vi "Edit waveform read from MDO.vi"() -> ()   [LabVIEW 2020]
uses:
  <vilib>/Utility/file.llb/Write Delimited Spreadsheet (DBL).vi
panel:
  in  "file (use dialog) in":path
  out "Array":dbl[][](array[numeric])
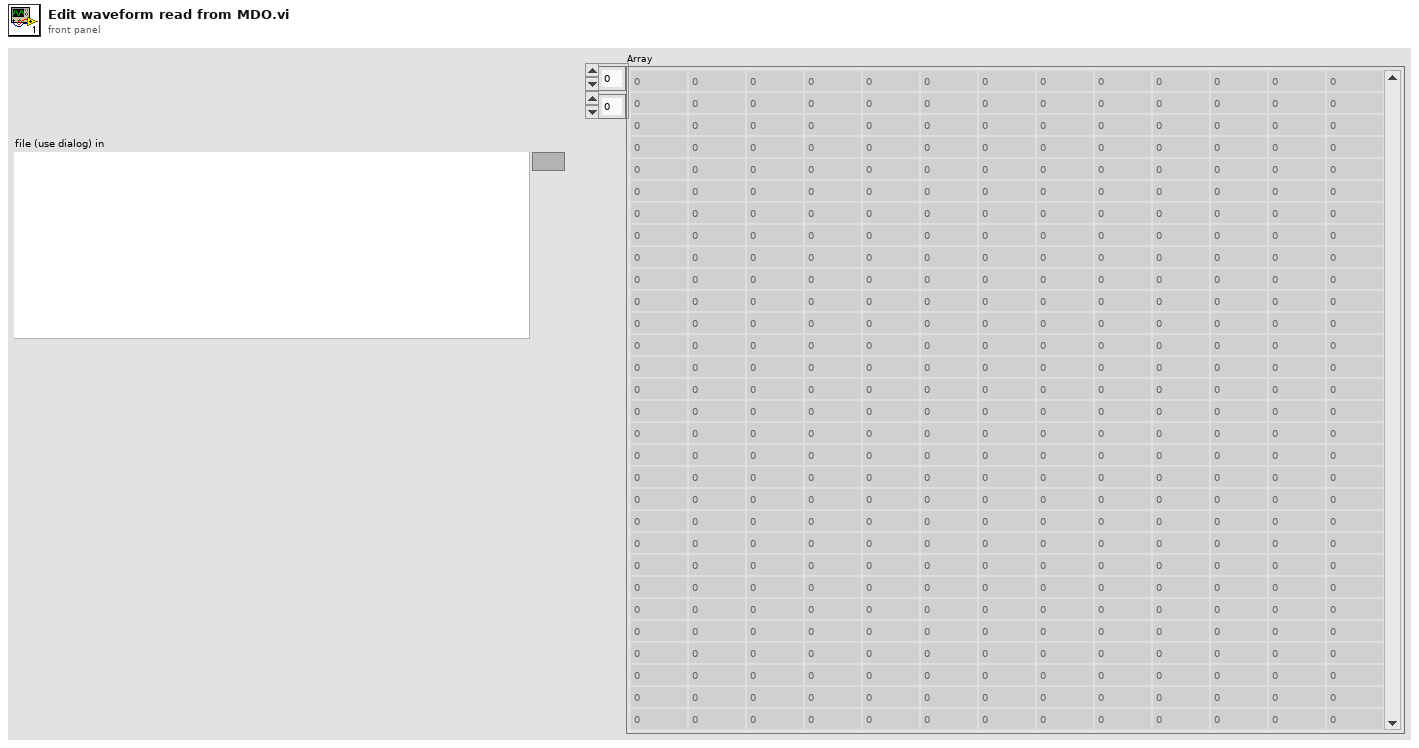
[diagram p1: front panel]
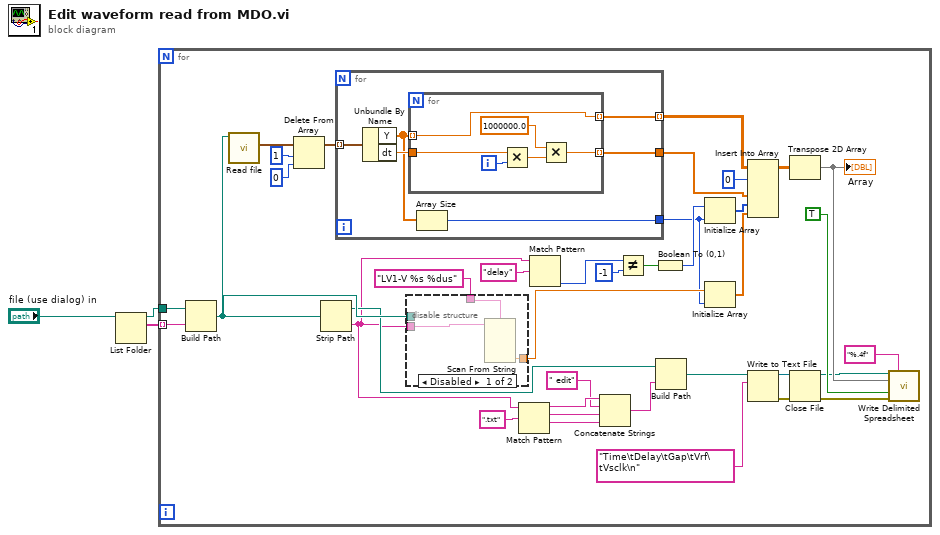
[diagram p0: block diagram]
diagram:
  n1 = List Folder(path="file (use dialog) in") -> (path out=w2:path, filenames=w1:string[])  [unwired: 3 in, 2 out]
  n2 = for {
    tunnel: w2 -> [w16]
    tunnel: w1 -> [w15] mode=indexing
    n3 = Build Path(base path=w16, name or relative path=w15) -> (appended path=w14:path)
    n4 = call "Read file.vi"("file (use dialog) in"=w14) -> ("Waveform Array"=w37:waveform(dbl)[])  [unwired: 7 in, 3 out]
    n5 = Delete From Array(array=w37, length=1, index=0) -> (array with subset deleted=w36:waveform(dbl)[])  [unwired: 1 out]
    n6 = Strip Path(path=w14) -> (stripped path=w5:path, name=w4:string)
    n7 = for {
      tunnel: w36 -> [w50] mode=indexing
      tunnel: [w48] -> w41 mode=indexing
      tunnel: [w47] -> w40
      tunnel: [w45] -> w8
      n8 = Unbundle By Name(w50) -> ("Y"=w46:dbl[], "dt"=w49:dbl)
      n9 = for {
        tunnel: w46 -> [w54] mode=indexing
        tunnel: w49 -> [w55]
        tunnel: [w54] -> w48 mode=indexing
        tunnel: [w51] -> w47 mode=indexing
        i -> [w56]
        n10 = Multiply(x=w55, y=w56) -> (x*y=w53:dbl)
        n11 = Multiply(x=1000000.0, y=w53) -> (x*y=w51:dbl)
      }
      n12 = Array Size(array=w46) -> (size(s)=w45:i32)
    }
    n13 = disable-structure shown="Disabled" {
      disable-tunnel: "LV1-V %s %dus" ("format string") -> [w44 _]
      disable-tunnel: [w43 _] -> w24
      disable-tunnel: w14 -> [_ _]
      disable-tunnel: w4 -> [w42 _]
      frame Disabled {
        n14 = Scan From String(format string=w44, input string=w42) -> (output 2=w43:dbl)  [unwired: 5 in, 3 out]
      }
      frame Enabled {
      }
    }
    n15 = Match Pattern(string=w4, regular expression=".txt") -> (before substring=w29:string, match substring=w28:string, after substring=w30:string)  [unwired: 1 in, 1 out]
    n16 = Match Pattern(string=w4, regular expression="delay") -> (offset past match=w12:i32)  [unwired: 1 in, 3 out]
    n17 = Concatenate Strings(w29, " edit" ("string"), w28, w30) -> (w26:string)
    n18 = Not Equal?(x=w12, y=-1) -> (x != y?=w10:bool)
    n19 = Boolean To (0,1)(Boolean=w10) -> (0, 1=w9:i16)
    n20 = Build Path(base path=w5, name or relative path=w26) -> (appended path=w19:path)
    n21 = Initialize Array(w9, w8) -> (w7:i16[])
    n22 = Initialize Array(w24, w8) -> (w6:dbl[])
    n23 = Insert Into Array(array=w41, index (row)=0, new element #1=w40, new element #2=w7, new element #3=w6) -> (w38:dbl[][])  [unwired: 1 in]
    n24 = Write to Text File(file (use dialog)=w19, text="Time\tDelay\tGap\tVrf\tVsclk\n") -> (refnum out=w23:refnum<file>, error out=w22:errorcluster)  [unwired: 2 in, 1 out]
    n25 = Transpose 2D Array(2D array=w38) -> (transposed array=w33:dbl[][])
    "Array" <- w33
    n26 = Close File(refnum=w23, error in=w22) -> (path=w20:path, error out=w18:errorcluster)
    n27 = call-poly <vilib>:"Write Delimited Spreadsheet.vi"("file path (dialog if empty)"=w20, "format (%.3f)"="%.4f", "2D data"=w33, "append to file? (new file:F)"=TRUE, "error in (no error)"=w18) -> ()  [unwired: 9 in, 2 out]
  }
